vi "Create Relay List.vi"(11 "Channels (1-64)":u16) -> (3 "Relay List":string)   [LabVIEW 2020, in "slsc-switch-benchmarks.lvlib"]
uses:
  slsc-switch-benchmarks.lvlib
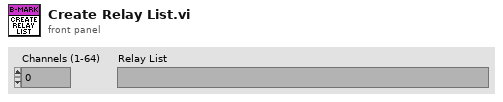
[diagram p1: front panel]
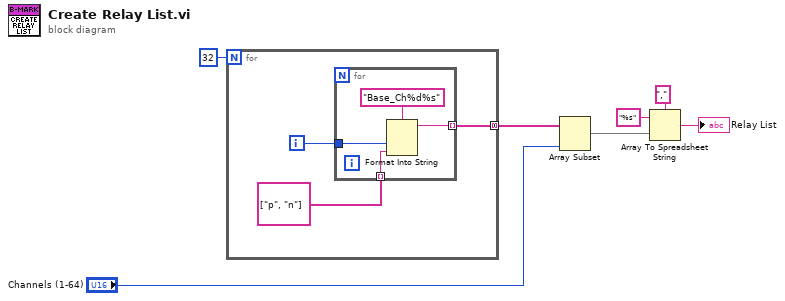
[diagram p0: block diagram]
diagram:
  n1 = for {
    N: 32 -> [_]
    tunnel: [w8] -> w2 mode=concatenating
    i -> [w10]
    n2 = for {
      tunnel: w10 -> [w13]
      tunnel: string[] ["p", "n"] -> [w12] mode=indexing
      tunnel: [w11] -> w8 mode=indexing
      n3 = Format Into String(format string="Base_Ch%d%s", w13, w12) -> (resulting string=w11:string)  [unwired: 2 in, 1 out]
    }
  }
  n4 = Array Subset(array=w2, length="Channels (1-64)") -> (w4:string[])  [unwired: 1 in]
  n5 = Array To Spreadsheet String(delimiter (Tab)=",", array=w4, 3:"%s" ("format string")) -> (spreadsheet string=→"Relay List":string)
